vi "DFF.vi"(0 "System no.":i32=1 min=1 max=4 step=1, 2 "Axis":string[](array[string]), 3 "Factor":dbl[](array[numeric]) format="%.6f", 4 "No.of digits":i16=4, 5 "error in":errorcluster) -> (19 "error out":errorcluster)   [LabVIEW 2020]
doc: "Defines scale factor which is applied to the basic unit (default is 1). E.g., 25.4 changes the physical unit from mm to inches. No. of digits is the number of digits after the decimal point in the factor value(s) that will be sent.\nExample: The physical unit is mm and the scale factor is 1. The current position of a stage is 12. Now the scale factor is set to 3 with DFF. Reading the position gives 4 as result. A relative move of 1.5 causes the stage to move 4.5 mm.\n\nAll systems: Factor can only be positive"
panel:
  # "Defines scale factor, e.g. 25.4 sets the logical unit to inches."
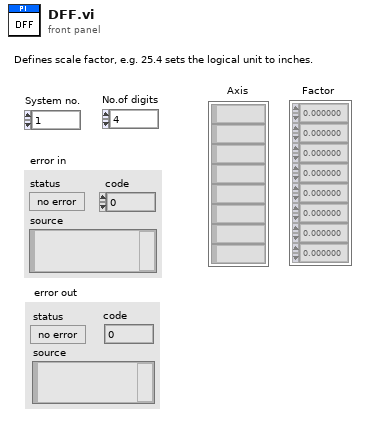
[diagram p1: front panel]
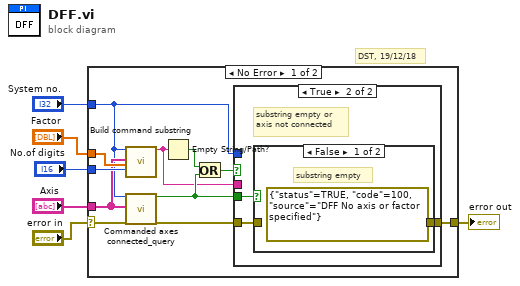
[diagram p0: block diagram]
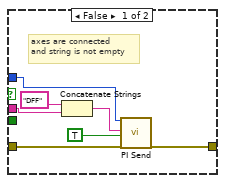
[diagram p2: hidden frame]
diagram:
  # "DST, 19/12/18"
  n1 = case shown="No Error" "error in" {
    selector: "error in" -> [w7 w30]
    tunnel: [w17 w30] -> w6
    tunnel: "Factor" -> [w16 _]
    tunnel: "No.of digits" -> [w15 _]
    tunnel: "System no." -> [w12 _]
    tunnel: "Axis" -> [w13 _]
    frame No Error {
      n2 = call "Build command substring.vi"("System no."=w12, "Affected axes"=w13, "Parameters"=w16, "No. of digits"=w15) -> ("Command substring"=w8:string)  [unwired: 3 in, 12 out]
      n3 = call "Commanded axes connected_query.vi"("System no."=w12, "Commanded axes"=w13, "error in"=w7) -> ("Controller error"=w10:bool, "error out"=w14:errorcluster)  [unwired: 1 in, 14 out]
      n4 = Empty String/Path?(string/path=w8) -> (empty?=w9:bool)
      n5 = Or(x=w9, y=w10) -> (x .or. y?=w11:bool)
      n6 = case shown="True" w11 {
        tunnel: w8 -> [w23 _]
        tunnel: [w19 w27] -> w17
        tunnel: w14 -> [w20 w25]
        tunnel: w10 -> [_ w26]
        tunnel: w12 -> [w18 _]
        frame False {
          # "axes are connected \nand string is not empty"
          n7 = Concatenate Strings("DFF", w23) -> (w21:string)
          n8 = call "PI Send.vi"("System no."=w18, "String to send"=w21, "Attach termination char.?"=TRUE ("Attach Linefeed?"), "error in"=w20) -> ("error out"=w19:errorcluster)  [unwired: 2 in, 13 out]
        }
        frame True {
          # "substring empty or \naxis not connected"
          n9 = case shown="False" w26 {
            tunnel: [errorcluster {"status"=TRUE, "code"=100, "source"="DFF No axis or factor specified"} ("error out") w29] -> w27
            tunnel: w25 -> [_ w29]
            frame False {
              # "substring empty"
            }
            frame True {
              # "commanded axis \nnot connected"
            }
          }
        }
      }
    }
    frame Error {
    }
  }
  "error out" <- w6
